vi "Test Multiple Write_Read.vi"(8 "error in (no error)":errorcluster, 11 "Scalar Channels Testing in":refnum<class "Scalar Channels Testing.lvclass">) -> (0 "error out":errorcluster, 3 "Scalar Channels Testing out":refnum<class "Scalar Channels Testing.lvclass">)   [LabVIEW 2019, in "Scalar Channels Testing.lvclass"]
uses:
  Scalar Channels Testing.lvclass
  C:/Program Files (x86)/National Instruments/LabVIEW 2019/vi.lib/NI/NI VeriStand Development Tools/NI Veristand Test Utilities/VeriStandTestCase/VeriStandTestCase.lvclass
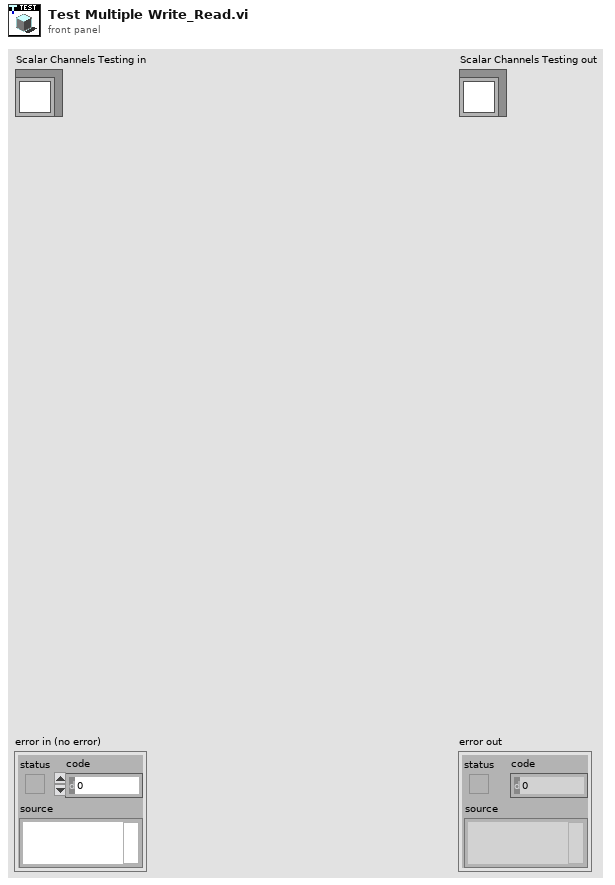
[diagram p1: front panel]
types:
  T1 = typedef "NI_VS Workspace ExecutionAPI.lvlib/WorkspaceAPI.ctl" = refnum<k24>
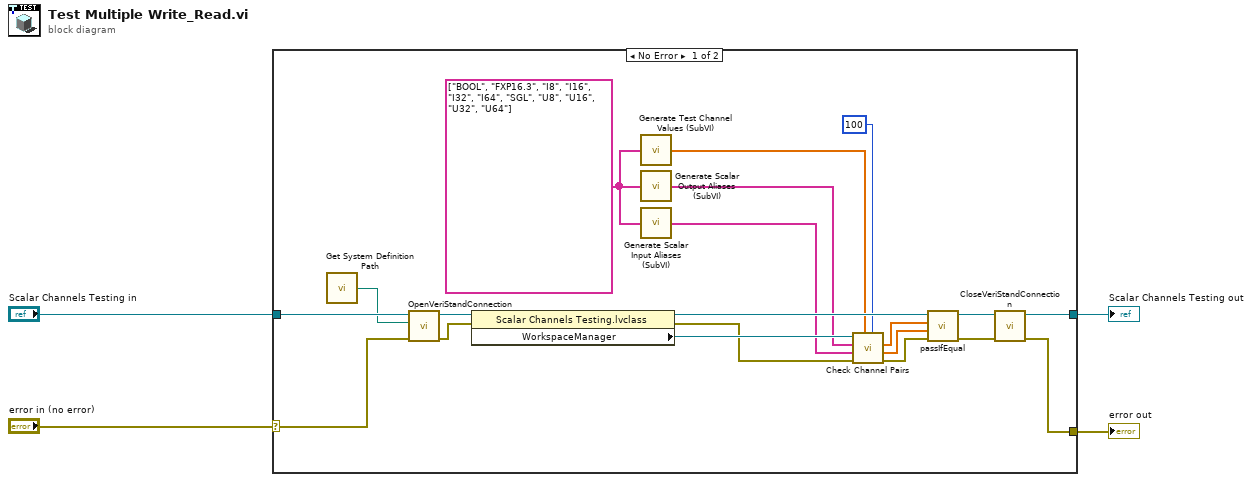
[diagram p0: block diagram]
diagram:
  n1 = case shown="No Error" "error in (no error)" {
    selector: "error in (no error)" -> [w22 w26]
    tunnel: [w21 w26] -> w3
    tunnel: [w23 w25] -> w1
    tunnel: "Scalar Channels Testing in" -> [w24 w25]
    frame No Error {
      w16 = string[] ["BOOL", "FXP16.3", "I8", "I16", "I32", "I64", "SGL", "U8", "U16", "U32", "U64"]
      n2 = call "Get System Definition Path.vi"() -> ("System Definition path"=w20:path)
      n3 = call-dynamic "OpenVeriStandConnection.vi"("error in (no error)"=w22, "System Definition File"=w20, "VeriStand Test Case in"=w24) -> ("error out"=w19:errorcluster, "VeriStand Test Case out"=w18:refnum<class "Scalar Channels Testing.lvclass">)  [unwired: 6 in, 1 out]
      n4 = property class="Scalar Channels Testing.lvclass"(reference=w18, error in=w19) -> (reference out=w14:refnum<class "Scalar Channels Testing.lvclass">, error out=w6:errorcluster, "WorkspaceManager"=w15:T1)
      n5 = call "Generate Test Channel Values (SubVI).vi"("Aliases in"=w16) -> ("Test Channel Values out"=w7:dbl[])
      n6 = call "Generate Scalar Output Aliases (SubVI).vi"("Aliases Seed"=w16) -> ("Scalar Output Aliases"=w11:string[])
      n7 = call "Generate Scalar Input Aliases (SubVI).vi"("Aliases Seed"=w16) -> ("Scalar Input Aliases"=w10:string[])
      n8 = call "Check Channel Pairs.vi"("milliseconds to wait"=u32 100, "Test Values"=w7, "error in (no error)"=w6, "Scalar Input Aliases"=w10, "Scalar Output Aliases"=w11, ".NET Refnum in"=w15) -> ("error out"=w13:errorcluster, "Input Scalar Channel Values"=w8:dbl[], "Output Scalar Channel Values"=w9:dbl[])  [unwired: 2 in, 1 out]
      n9 = call-dynamic "passIfEqual.vi"("error in (no error)"=w13, "y"=w8, "x"=w9, "TestCase in"=w14) -> ("error out"=w17:errorcluster, "TestCase out"=w12:refnum<class "Scalar Channels Testing.lvclass">)  [unwired: 6 in]
      n10 = call-dynamic "CloseVeriStandConnection.vi"("error in (no error)"=w17, "VeriStand Test Case in"=w12) -> ("error out"=w21:errorcluster, "VeriStand Test Case out"=w23:refnum<class "Scalar Channels Testing.lvclass">)  [unwired: 8 in]
    }
    frame Error {
    }
  }
  "error out" <- w3
  "Scalar Channels Testing out" <- w1
